vi "DSF.Engine.Memory.Cache.Plugin.Initialize.vi"(8 "error in (no error)":errorcluster, 10 "Device Ref in":T1=18446744073709551615 format="%.0x", 11 "Plugin Cache in":refnum<class "DSF.Engine.Memory.Cache.Plugin.lvclass">) -> (0 "error out":errorcluster, 3 "Plugin Cache out":refnum<class "DSF.Engine.Memory.Cache.Plugin.lvclass">)   [LabVIEW 2016, in "DSF.Engine.lvlib" / "DSF.Engine.Memory.Cache.Plugin.lvclass"]
uses:
  DSF.Engine.Memory.Cache.Plugin.lvclass
  <vilib>/NI Veristand/Custom Device API/Custom Device Item Ref.ctl
  DSF.Engine.Memory.Cache.Plugin.lvclass/DSF.Engine.Memory.Cache.Plugin.ctl
  DSF.Engine.Memory.Cache.Transfer Group.lvclass/DSF.Engine.Memory.Cache.Transfer Group.ctl
  DSF.Engine.Memory.Cache.Transfer.lvclass/DSF.Engine.Memory.Cache.Transfer.ctl
  Shared/Classes/Transfer/DSF.Shared.Configuration.Transfer.lvclass/DSF.Shared.Configuration.Transfer.ctl
  DSF.Engine.Memory.Cache.Transfer Group.Set Transfer Caches.vi
  DSF.Engine.Memory.Cache.Transfer.Initialize.vi
  DSF.Engine.Memory.Cache.Transfer Group.Get Transfer Caches.vi
  DSF.Engine.Memory.Cache.Transfer.Initialize Buffer.vi
  DSF.Engine.Memory.Cache.Transfer.Initialize Channels Pointer.vi
  Shared/Classes/Transfer/DSF.Shared.Configuration.Transfer.Required Buffer Size.vi
  DSF.Engine.Memory.Cache.Transfer.Set Buffer.vi
  DSF.Engine.Memory.Cache.Transfer.Get Configuration.vi
  DSF.Engine.Memory.Cache.Transfer.Set VS Channels Pointer.vi
  Pointer/DSF.Engine.Memory.Pointer.VS Channels.New.vi
  Shared/Classes/Transfer/DSF.Shared.Configuration.Transfer.Get Block Descriptors.vi
  Shared/Classes/Transfer/DSF.Shared.Configuration.Transfer.Get Channel Count.vi
  Shared/Classes/Transfer/DSF.Shared.Configuration.Transfer.Get Access Mode.vi
  Shared/VIs/DSF.Shared.Data Type.Sizeof.1D.vi
  Pointer/DSF.Engine.Memory.Pointer.VS Channels.Data Ref to Pointer.vi
  Shared/Classes/Transfer/DSF.Shared.Configuration.Transfer.Get Channel Descriptors.vi
  Shared/Classes/Transfer/DSF.Shared.Configuration.Transfer.Get Direction.vi
  Shared/VIs/DSF.Shared.Data Type.Sizeof.vi
  Pointer/DSF.Engine.Memory.Pointer.VS Channels.lvclass
  C:/Git/Sourcetree/DSF/Source/Submodules/Memory/Source/Classes/External/Memory.Pointer.External.lvclass
  Submodules/Memory/Source/Classes/External/Memory.Pointer.External.Encapsulate.vi
  <vilib>/NI Veristand/Custom Device API/Global Data Refs.vi
  <vilib>/NI Veristand/Custom Device API/NI VeriStand - Get Channel Data Reference.vi
  Buffer/DSF.Engine.Memory.Buffer.New.vi
  DSF.Engine.Memory.Cache.Transfer Group.lvclass
  <vilib>/NI Veristand/Custom Device API/Custom Device API.lvlib
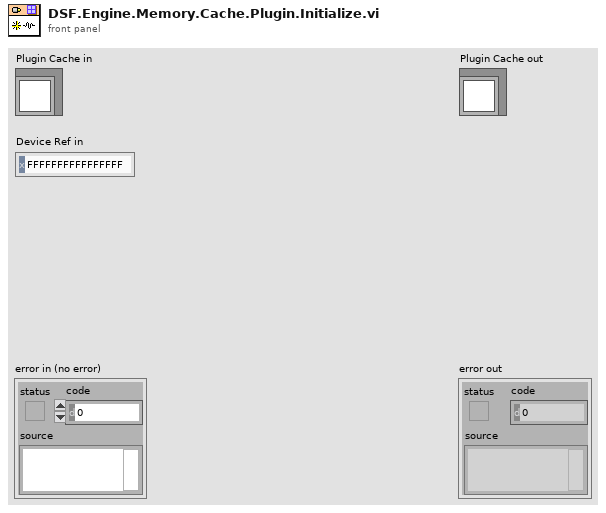
[diagram p1: front panel]
types:
  T1 = typedef "Custom Device API.lvlib/Custom Device Item Ref.ctl" = u64
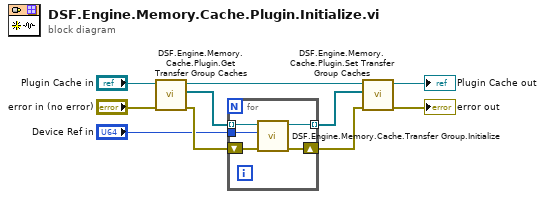
[diagram p0: block diagram]
diagram:
  n1 = call "DSF.Engine.Memory.Cache.Plugin.Get Transfer Group Caches.vi"("error in (no error)"="error in (no error)", "Plugin Cache in"="Plugin Cache in") -> ("error out"=w5:errorcluster, "Transfer Group Caches"=w4:refnum<class "DSF.Engine.Memory.Cache.Transfer Group.lvclass">[], "Plugin Cache out"=w9:refnum<class "DSF.Engine.Memory.Cache.Plugin.lvclass">)  [unwired: 7 in]
  n2 = for {
    tunnel: [w15] -> w8 mode=indexing
    tunnel: "Device Ref in" -> [w11]
    shift-right: [w14] -> w10
    shift-left: w5 -> [w13]
    tunnel: w4 -> [w12] mode=indexing
    n3 = call "DSF.Engine.Memory.Cache.Transfer Group.Initialize.vi"("error in (no error)"=w13, "Device Ref in"=w11, "Transfer Group Cache in"=w12) -> ("error out"=w14:errorcluster, "Transfer Group Cache out"=w15:refnum<class "DSF.Engine.Memory.Cache.Transfer Group.lvclass">)  [unwired: 7 in]
  }
  n4 = call "DSF.Engine.Memory.Cache.Plugin.Set Transfer Group Caches.vi"("error in (no error)"=w10, "Transfer Group Caches"=w8, "Plugin Cache in"=w9) -> ("error out"=→"error out":errorcluster, "Plugin Cache out"=→"Plugin Cache out":refnum<class "DSF.Engine.Memory.Cache.Plugin.lvclass">)  [unwired: 7 in]
